vi "InsertDevData.vi"(8 "错误输入":errorcluster, 9 "DevnASData":T1, 10 "选定检测区域":string, 11 "date/time string":string) -> (0 "错误输出":errorcluster, 1 "elecNum":i32, 2 "数据采集模块地址":string, 3 "detec_electrode_name":string)   [LabVIEW 2014, in "DataBase.lvlib"]
uses:
  DataBase.lvlib
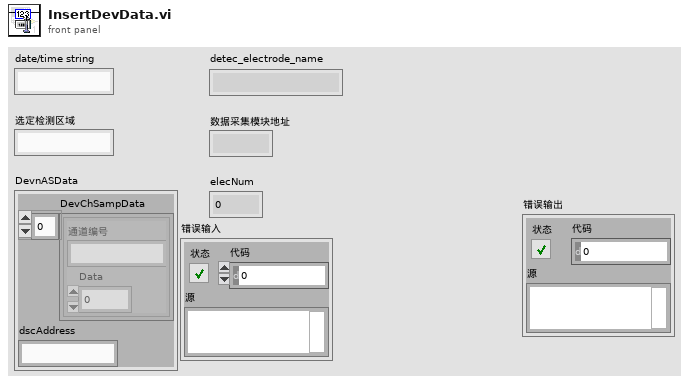
[diagram p1: front panel]
types:
  T1 = cluster{"DevChSampData":cluster{"通道编号":string, "Data":dbl}[], "dscAddress":string}
  T2 = cluster{string, "date/time string":string, "detec_electrode_name":string, "electrodes_map_x":string, "electrodes_map_y":string, string}
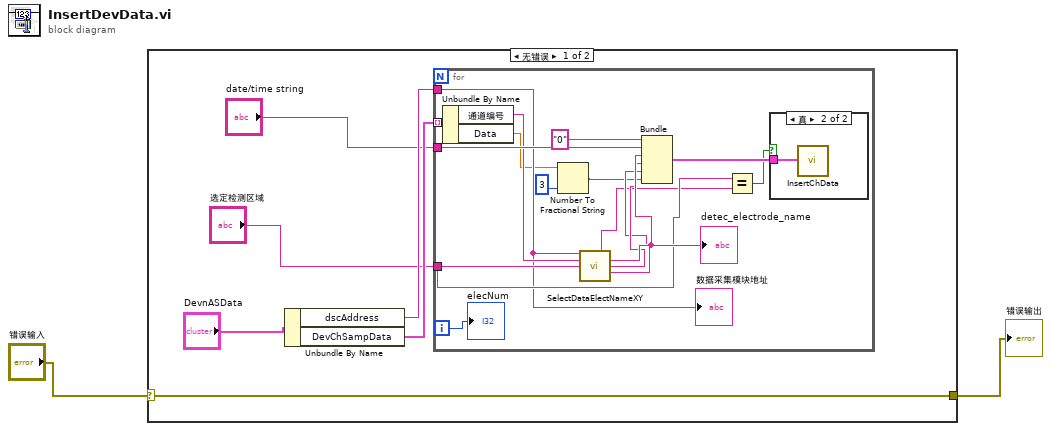
[diagram p0: block diagram]
diagram:
  n1 = case shown="无错误" "错误输入" {
    selector: "错误输入" -> [w3 w26]
    tunnel: [w3 w26] -> w1
    frame No Error {
      n2 = Unbundle By Name("DevnASData") -> ("dscAddress"=w8:string, "DevChSampData"=w7:cluster{"通道编号":string, "Data":dbl}[])
      n3 = for {
        tunnel: "date/time string" -> [w24]
        tunnel: w7 -> [w19] mode=indexing
        tunnel: "选定检测区域" -> [w15]
        tunnel: w8 -> [w12]
        i -> [w16]
        n4 = Unbundle By Name(w19) -> ("通道编号"=w18:string, "Data"=w11:dbl)
        n5 = Number To Fractional String(number=w11, precision (6)=i16 3 ("精度(6)")) -> (F-format string=w10:string)  [unwired: 2 in]
        n6 = call "SelectDataElectNameXY.vi"("dsc_board_address"=w12, "elec_num"=w18, "area_name"=w15) -> ("area_name"=w14:string, "detec_electrode_name"=w22:string, "electrodes_map_x"=w21:string, "electrodes_map_y"=w20:string)  [unwired: 7 in, 2 out]
        "detec_electrode_name" <- w22
        n7 = Bundle("0", "date/time string"=w24, "detec_electrode_name"=w22, "electrodes_map_x"=w21, "electrodes_map_y"=w20, w10) -> (w17:T2)  [unwired: 1 in]
        n8 = Equal?(x=w15, y=w14) -> (x = y?=w13:bool)
        n9 = case shown="真" w13 {
          tunnel: w17 -> [_ w25]
          frame False {
          }
          frame True {
            n10 = call "InsertChData.vi"("检测数据"=w25) -> ()  [unwired: 10 in, 1 out]
          }
        }
        "数据采集模块地址" <- w12
        "elecNum" <- w16
      }
    }
    frame Error {
    }
  }
  "错误输出" <- w1
